vi "Convert Data and Overwrite Original File.vi"(8 "error in":errorcluster, 11 "refnum in":refnum<file>) -> (0 "error out":errorcluster, 3 "refnum out":refnum<file>)   [LabVIEW 2017]
uses:
  <vilib>/Analysis/NI_AALBase.lvlib
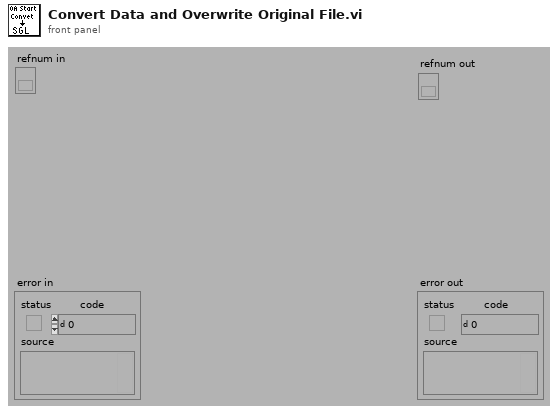
[diagram p1: front panel]
types:
  T1 = cluster{"name":string, "multiplier":sgl, "offset":sgl, "sensor sensitivity (mV/EU)":dbl, "engineering units":enum16{"custom...", "V", "Pa", "g", "m/s^2", "m/s", "m", "in/s^2", "in/s", "in"}}[]
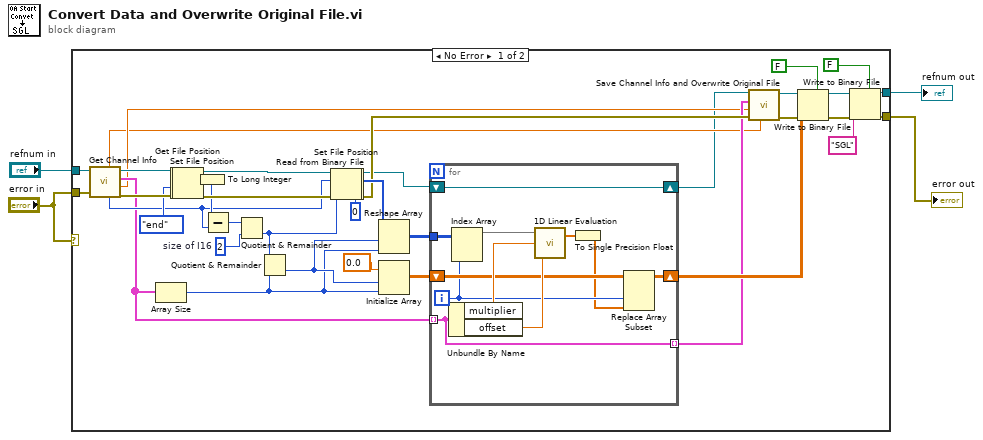
[diagram p0: block diagram]
diagram:
  n1 = case shown="No Error" "error in" {
    tunnel: "refnum in" -> [w45 w58]
    tunnel: "error in" -> [w34 w57]
    tunnel: [w14 w58] -> w3
    tunnel: [w13 w57] -> w2
    frame No Error {
      w37 = 2  # size of I16
      n2 = call <vilib>:"Get Channel Info.vi"("error in"=w34, "refnum in"=w45) -> ("error out"=w41:errorcluster, "time"=w20:dbl, "channel information"=w22:T1, "dup refnum"=w42:refnum<file>, "data offset"=w35:i32, "Sample rate"=w19:sgl)  [unwired: 4 in]
      n3 = Array Size(array=w22) -> (size(s)=w29:i32)
      n4 = Set File Position(refnum=w42, from (0:start)=enum16{"start", "end", "current"}."end" ("pos mode (0:2)"), error in=w41) -> (refnum out=w7:refnum<file>, error out=w6:errorcluster)  [unwired: 1 in]
      n5 = Get File Position(4:w6, 7:w7) -> (0:w44:errorcluster, 2:w5:i64, 3:w43:refnum<file>)
      n6 = To Long Integer(number=w5) -> (32bit integer=w39:i32)
      n7 = Subtract(x=w39, y=w35) -> (x-y=w38:i32)
      n8 = Quotient & Remainder(x=w38, y=w37) -> (floor(x/y)=w36:i32)  [unwired: 1 out]
      n9 = Quotient & Remainder(x=w36, y=w29) -> (floor(x/y)=w30:i32)  [unwired: 1 out]
      n10 = Set File Position(offset (in bytes) (0)=w35, refnum=w43, error in=w44) -> (refnum out=w9:refnum<file>, error out=w8:errorcluster)  [unwired: 1 in]
      n11 = Read from Binary File(5:i16 0, 8:w8, 10:w36, 11:w9) -> (0:w23:errorcluster, 2:w32:i16[], 3:w18:refnum<file>)  [unwired: 2 in, 1 out]
      n12 = Reshape Array(w32, w30, w29) -> (w31:i16[][])
      n13 = Initialize Array(sgl 0.0 ("element"), w30, w29) -> (w27:sgl[][])
      n14 = for {
        tunnel: w31 -> [w56]
        tunnel: w22 -> [w47] mode=indexing
        shift-right: [w48] -> w26
        shift-left: w27 -> [w51]
        tunnel: [w47] -> w21 mode=indexing
        shift-right: [w46] -> w17
        shift-left: w18 -> [w46]
        i -> [w50]
        n15 = Unbundle By Name(w47) -> ("multiplier"=w54:sgl, "offset"=w53:sgl)
        n16 = Index Array(array=w56, index (col)=w50) -> (element=w55:i16[])  [unwired: 1 in]
        n17 = call <vilib>:"1D Linear Evaluation.vi"("offset"=w53, "scale"=w54, "X"=w55) -> ("Y[i]=X[i]*a+b"=w52:dbl[])  [unwired: 1 out]
        n18 = To Single Precision Float(number=w52) -> (single precision float=w49:sgl[])
        n19 = Replace Array Subset(array=w51, new element=w49, index (col)=w50) -> (w48:sgl[][])  [unwired: 1 in]
      }
      n20 = call <vilib>:"Save Channel Info and Overwrite Original File.vi"("Sample rate"=w19, "error in"=w23, "time"=w20, "channel info"=w21, "refnum in"=w17) -> ("error out"=w24:errorcluster, "refnum out"=w25:refnum<file>)  [unwired: 5 in]
      n21 = Write to Binary File(file (use dialog)=w25, data=w26, error in=w24, 5:FALSE ("prepend array or string size? (T)")) -> (refnum out=w16:refnum<file>, error out=w15:errorcluster)  [unwired: 2 in, 1 out]
      n22 = Write to Binary File(file (use dialog)=w16, data="SGL", error in=w15, 5:FALSE ("prepend array or string size? (T)")) -> (refnum out=w14:refnum<file>, error out=w13:errorcluster)  [unwired: 2 in, 1 out]
    }
    frame Error {
    }
  }
  "refnum out" <- w3
  "error out" <- w2
